vi "Calculate Velocity.vi"(8 "error in":errorcluster, 10 "Mixing Time":timestamp, 11 "Potting Parameters":T1) -> (0 "error out":errorcluster, 3 "Velocity":dbl)   [LabVIEW 2017]
uses:
  Config Manager Class/Type Definitions/Potting Parameters.ctl
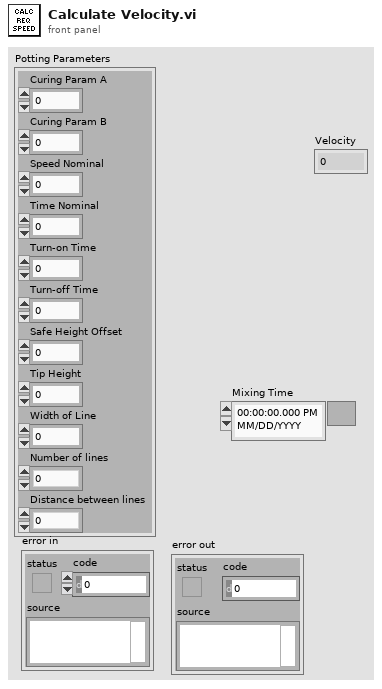
[diagram p1: front panel]
types:
  T1 = typedef "Potting Parameters.ctl" = cluster{"Curing Param A":dbl, "Curing Param B":dbl, "Speed Nominal":dbl, "Time Nominal":dbl, "Turn-on Time":dbl, "Turn-off Time":dbl, "Safe Height Offset":dbl, "Tip Height":dbl, "Width of Line":dbl, "Number of lines":dbl, "Distance between lines":dbl}
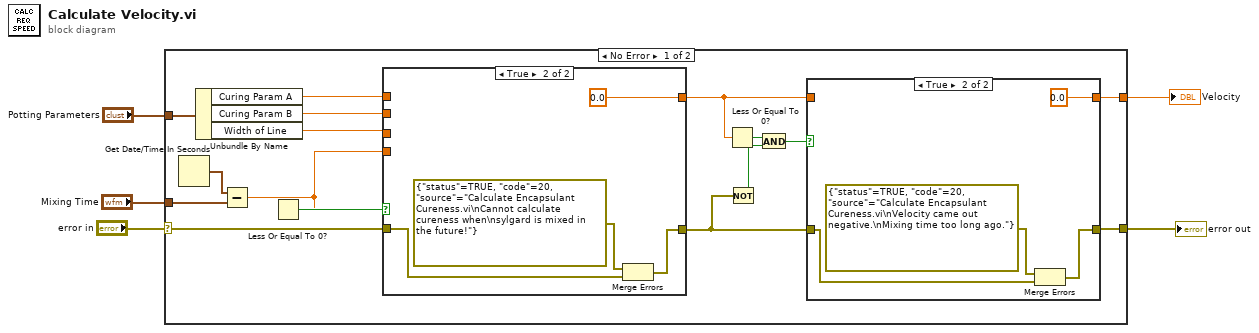
[diagram p0: block diagram]
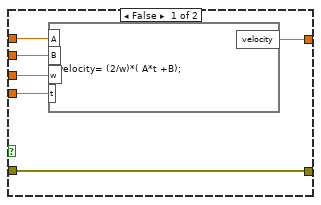
[diagram p3: hidden frame]
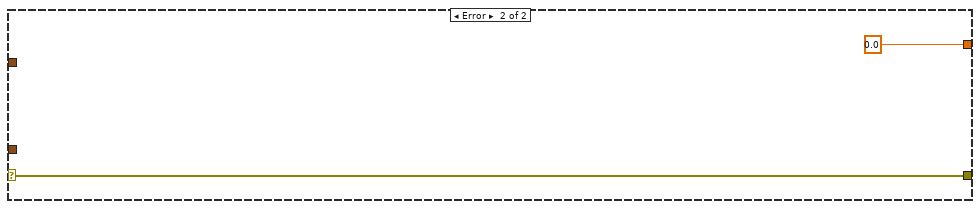
[diagram p4: hidden frame]
diagram:
  n1 = case shown="No Error" "error in" {
    selector: "error in" -> [w17 w39]
    tunnel: "Potting Parameters" -> [w21 _]
    tunnel: "Mixing Time" -> [w20 _]
    tunnel: [w15 0.0 ("cureness")] -> w3
    tunnel: [w16 w39] -> w1
    frame No Error {
      n2 = Get Date/Time In Seconds() -> (seconds since 1Jan1904=w19:timestamp)
      n3 = Unbundle By Name(w21) -> ("Curing Param A"=w11:dbl, "Curing Param B"=w13:dbl, "Width of Line"=w6:dbl)
      n4 = Subtract(x=w19, y=w20) -> (x-y=w12:dbl)
      n5 = Less Or Equal To 0?(x=w12) -> (x <= 0?=w18:bool)
      n6 = case shown="True" w18 {
        tunnel: w17 -> [w33 w37]
        tunnel: [w33 w35] -> w10
        tunnel: [w29 0.0 ("cureness")] -> w14
        tunnel: w13 -> [w31 _]
        tunnel: w12 -> [w30 _]
        tunnel: w11 -> [w32 _]
        tunnel: w6 -> [w28 _]
        frame False {
          n7 = formula code="velocity= (2/w)*( A*t +B);"("A"=w32, "B"=w31, "t"=w30, "w"=w28) -> ("velocity"=w29:dbl)
        }
        frame True {
          n8 = Merge Errors(errorcluster {"status"=TRUE, "code"=20, "source"="Calculate Encapsulant Cureness.vi\nCannot calculate cureness when\nsylgard is mixed in the future!"} ("error constant"), w37) -> (w35:errorcluster)
        }
      }
      n9 = Less Or Equal To 0?(x=w14) -> (x <= 0?=w8:bool)
      n10 = Not(x=w10) -> (.not. x?=w9:bool)
      n11 = And(x=w8, y=w9) -> (x .and. y?=w7:bool)
      n12 = case shown="True" w7 {
        tunnel: w10 -> [w23 w27]
        tunnel: [w23 w25] -> w16
        tunnel: [w22 0.0 ("cureness")] -> w15
        tunnel: w14 -> [w22 _]
        frame False {
        }
        frame True {
          n13 = Merge Errors(errorcluster {"status"=TRUE, "code"=20, "source"="Calculate Encapsulant Cureness.vi\nVelocity came out negative.\nMixing time too long ago."} ("error constant"), w27) -> (w25:errorcluster)
        }
      }
    }
    frame Error {
    }
  }
  "Velocity" <- w3
  "error out" <- w1
